vi "SET_ATTEN.vi"(0 "VISA resource name":refnum<visa-resource-name>, 11 "error in (no error)":errorcluster, 12 "Auto Mechanical Attenuation (T: Enable)":bool=TRUE, 13 "Att (dB)":u16(ring) items=["0"=0, "10"=10, "20"=20, "30"=30, "40"=40, "50"=50, "60"=60]) -> (4 "VISA resource name out":refnum<visa-resource-name>, 15 "error out":errorcluster)   [LabVIEW 2018]
doc: "Configures the vertical settings of the spectrum analyzer without Electrical Attenuation."
uses:
  Agilent MXA Series/Agilent MXA Series.lvlib
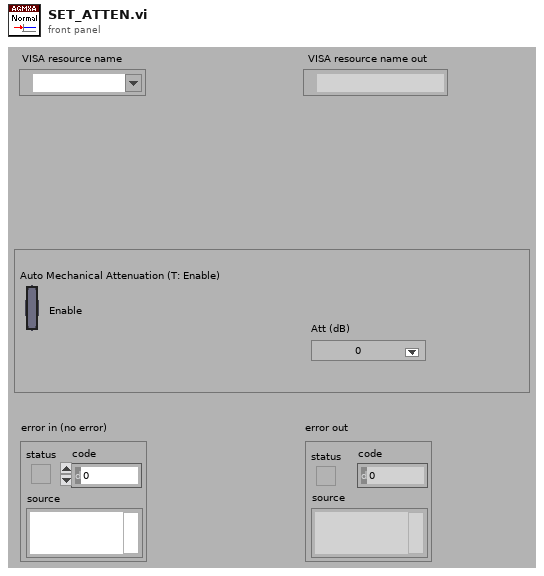
[diagram p1: front panel]
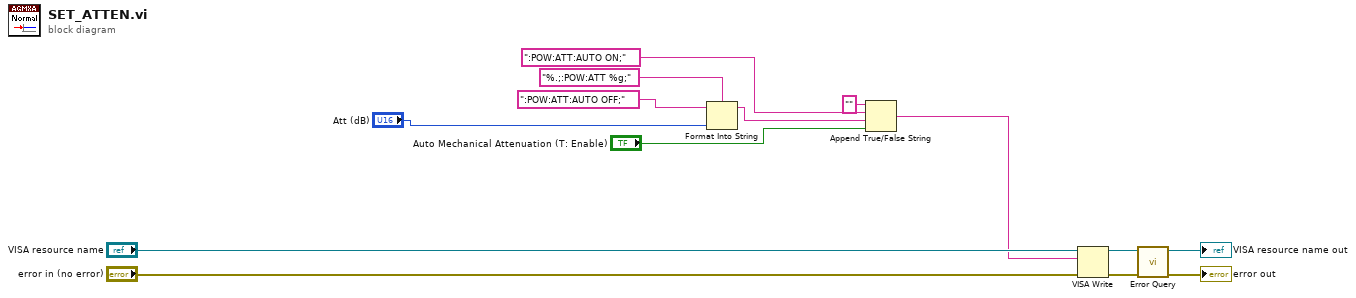
[diagram p0: block diagram]
diagram:
  n1 = Format Into String(format string="%.;:POW:ATT %g;", initial string=":POW:ATT:AUTO OFF;", "Att (dB)") -> (resulting string=w8:string)  [unwired: 1 in, 1 out]
  n2 = Append True/False String(1:"Auto Mechanical Attenuation (T: Enable)", 2:w8, 3:":POW:ATT:AUTO ON;" ("true string"), 4:"" ("string (\"\")")) -> (0:w3:string)
  n3 = VISA Write(VISA resource name="VISA resource name", write buffer=w3, error in (no error)="error in (no error)") -> (VISA resource name out=w14:refnum<visa-resource-name>, error out=w12:errorcluster)  [unwired: 1 out]
  n4 = call "Error Query.vi"("error in (no error)"=w12, "VISA resource name"=w14) -> ("error out"=→"error out":errorcluster, "VISA resource name out"=→"VISA resource name out":refnum<visa-resource-name>)  [unwired: 6 in, 2 out]
